vi "calibration.vi"() -> (0 "My Threshold":dbl=1.0)   [LabVIEW 2016]
panel:
  out "My Muscle Signal":dbl(graph)
  in  "Calibrate":bool
  in  "stop":bool
  # "Calibration Instruction:\n1.Keep your muscle relaxed. \n2.Press 'Calibrate' button to start.\n3.Keep your muscle relaxed and wait for around 5 seconds.\n4.Press 'Calibrate' button again to stop.\n5.You can repeat the process 2-4 again if you moved your mucle or the sensor during the calibration. \n6. Press the 'Exit' button when you are happy with your threshold."
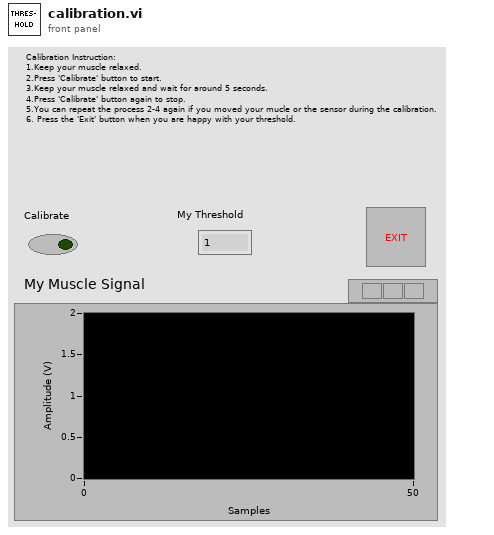
[diagram p1: front panel]
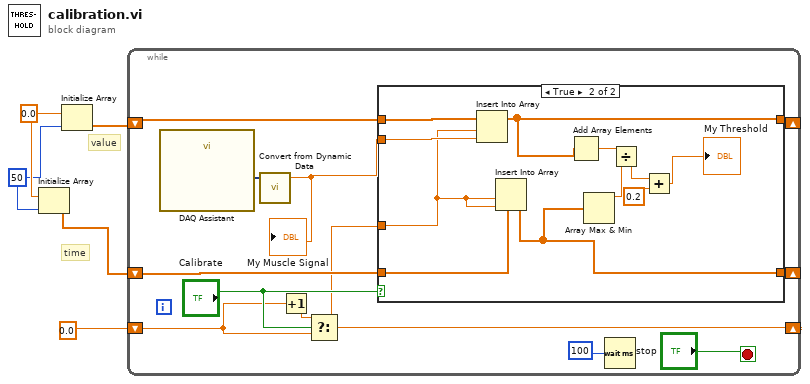
[diagram p0: block diagram]
diagram:
  w4 = 50 ("dimension size")
  w5 = 0.0 ("element")
  # "value"
  # "time"
  n1 = Initialize Array(w5, w4) -> (w2:dbl[])
  n2 = Initialize Array(w5, w4) -> (w3:dbl[])
  n3 = while {
    shift-right: [w11] -> _
    shift-left: w3 -> [w15]
    shift-right: [w10] -> _
    shift-left: w2 -> [w14]
    shift-right: [w7] -> _
    shift-left: 0.0 -> [w6]
    stop <- "stop" stop-if-true
    n4 = call "DAQ Assistant"() -> ("data"=w16:dynamicdata)  [unwired: 17 in, 2 out]
    n5 = call "Convert from Dynamic Data"("Dynamic Data Type"=w16) -> ("Scalar"=w12:dbl)  [unwired: 3 in]
    "My Muscle Signal" <- w12
    n6 = Increment(x=w6) -> (x+1=w8:dbl)
    n7 = Select(t=w8, s="Calibrate", f=w6) -> (s? t:f=w7:dbl)
    n8 = case shown="True" "Calibrate" {
      tunnel: w12 -> [_ w30]
      tunnel: w15 -> [w19 w29]
      tunnel: [w19 w24] -> w11
      tunnel: [w18 w25] -> w10
      tunnel: w14 -> [w18 w28]
      tunnel: w7 -> [_ w23]
      frame False {
      }
      frame True {
        n9 = Insert Into Array(array=w29, index=w23, new element=w30) -> (w24:dbl[])
        n10 = Insert Into Array(array=w28, index=w23, new element=w23) -> (w25:dbl[])
        n11 = Add Array Elements(numeric array=w24) -> (sum=w26:dbl)
        n12 = Array Max & Min(array=w25) -> (max value=w27:dbl)  [unwired: 3 out]
        n13 = Divide(x=w26, y=w27) -> (x/y=w20:dbl)
        n14 = Add(x=w20, y=0.2) -> (x+y=→"My Threshold":dbl)
      }
    }
    n15 = Wait (ms)(milliseconds to wait=u32 100) -> ()  [unwired: 1 out]
  }
